vi "Telescope Configure GUI.vi"(8 "error in (no error)":errorcluster, 10 "Telescope Name":string="Default", 11 "Telescope Simulator in":refnum<class "Telescope Simulator.lvclass">) -> (0 "error out":errorcluster, 3 "Telescope Simulator out":refnum<class "Telescope Simulator.lvclass">)   [LabVIEW 2021, in "Telescope Simulator.lvclass"]
uses:
  Telescope Simulator.lvclass
  Telescope Simulator.lvclass/Telescope Simulator.ctl
  Telescope.lvclass
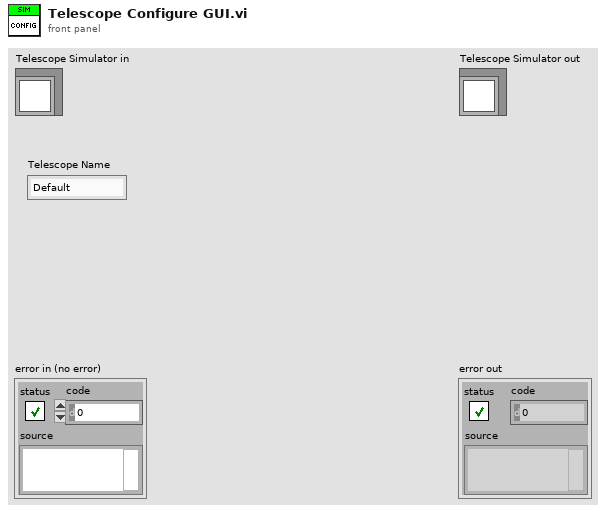
[diagram p1: front panel]
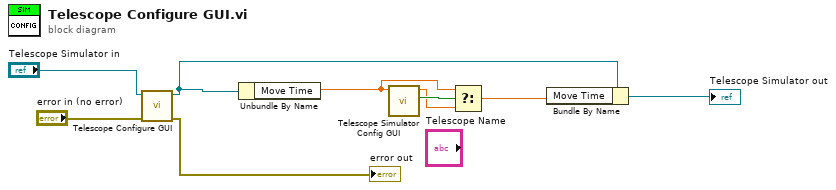
[diagram p0: block diagram]
diagram:
  n1 = call-parent "Telescope Configure GUI.vi"("error in (no error)"="error in (no error)", "Telescope in"="Telescope Simulator in") -> ("error out"=→"error out":errorcluster, "Telescope out"=w3:refnum<class "Telescope Simulator.lvclass">)  [unwired: 8 in]
  n2 = Unbundle By Name(w3) -> ("Move Time"=w5:dbl)
  n3 = call "Telescope Simulator Config GUI.vi"("Time to Move Between Positions"=w5) -> ("Cancelled"=w6:bool, "Time out"=w4:dbl)  [unwired: 9 in]
  n4 = Select(t=w5, s=w6, f=w4) -> (s? t:f=w2:dbl)
  n5 = Bundle By Name(cluster=w3, "Move Time"=w2) -> (→"Telescope Simulator out":refnum<class "Telescope Simulator.lvclass">)
